vi "AddClassPropertiesInline.vi"(9 "Count":i32, 11 "Math.lvclass":refnum<class "Math.lvclass">) -> (3 "Math.lvclass out":refnum<class "Math.lvclass">)   [LabVIEW 2016, in "Math.lvclass"]
uses:
  Math.lvclass
  Math.lvclass/Math.ctl
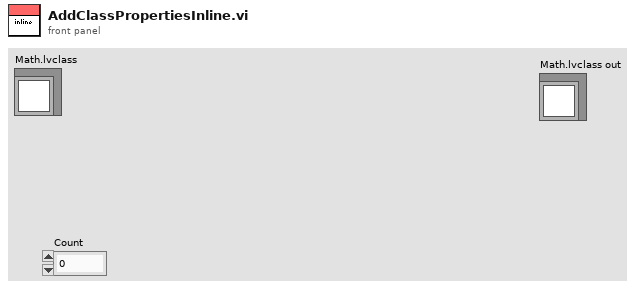
[diagram p1: front panel]
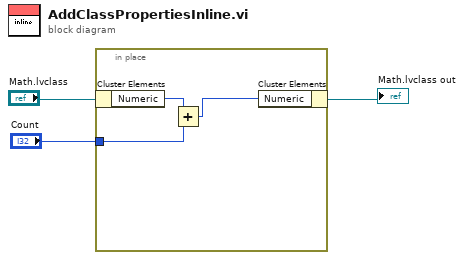
[diagram p0: block diagram]
diagram:
  n1 = in-place {
    in-place-border: "Count" -> [w5]
    n2 = in-place-cluster #1("Math.lvclass") -> ("Numeric"=w6:i32)
    n3 = Add(x=w6, y=w5) -> (x+y=w4:i32)
    n4 = in-place-cluster #1("Numeric"=w4) -> (→"Math.lvclass out":refnum<class "Math.lvclass">)
  }
